vi "calculate_checksum.vi"(10 "Byte array":u8[](array[numeric])) -> (2 "Checksum":u8)   [LabVIEW 2018]
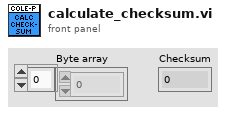
[diagram p1: front panel]
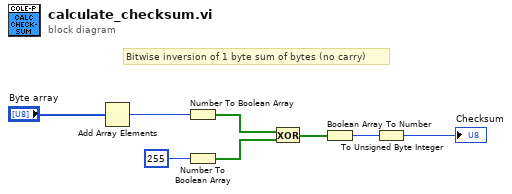
[diagram p0: block diagram]
diagram:
  # "Bitwise inversion of 1 byte sum of bytes (no carry)"
  n1 = Add Array Elements(numeric array="Byte array") -> (sum=w4:u8)
  n2 = Number To Boolean Array(number=w4) -> (Boolean array=w6:bool[])
  n3 = Number To Boolean Array(number=u8 255) -> (Boolean array=w7:bool[])
  n4 = Exclusive Or(1:w7, 2:w6) -> (0:w8:bool[])
  n5 = Boolean Array To Number(Boolean array=w8) -> (number=w2:u32)
  n6 = To Unsigned Byte Integer(number=w2) -> (unsigned 8bit integer=→"Checksum":u8)
